vi "Periodic Tasks.vi"(8 "error in":errorcluster) -> ()   [LabVIEW 2018]
doc: "This VI runs in parallel to other tasks. It can contain as many user-defined periodic loops as you need. These can carry out PID or other sorts of timed response."
uses:
  <vilib>/Rock Robotics/WPI/ThirdParty/Sensors/navX/_TypeDefs/FRIC_navX_DeviceNumbersTypeDef.ctl
  <vilib>/Rock Robotics/WPI/Relay/WPI_RelayValue.ctl
  <vilib>/Rock Robotics/WPI/DriverStation/WPI_DriverStationRobotMode2.ctl
  <vilib>/Rock Robotics/WPI/Utilities/WPI_GetSetVariantRefNum.vi
  Robot Global Data.vi
  <vilib>/Rock Robotics/Network Tables/NT Write Number.vi
  <vilib>/Rock Robotics/WPI/ThirdParty/Phoenix-LabVIEW/Motor Controller/Get/CTRE_Phoenix_MotorController_GetQuadratureData.vi
  <vilib>/Rock Robotics/WPI/ThirdParty/Sensors/navX/_Processing Loop/FRIC_navX_Internal_Serial_ProcessingLoop.vi
panel:
  out "Largeur Vision":dbl
  out "Gauche Droite Vision":dbl
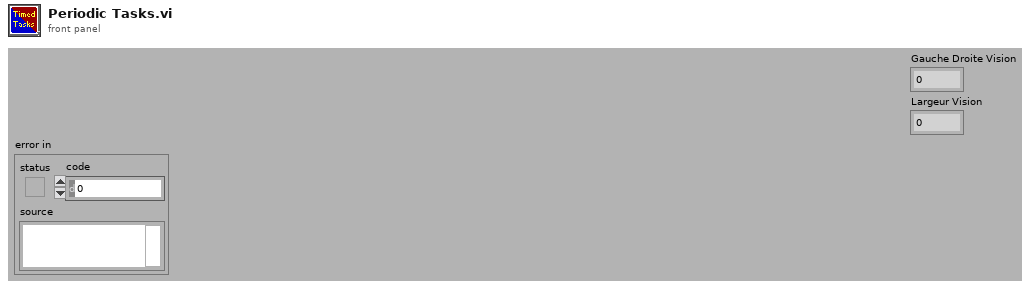
[diagram p1: front panel]
types:
  T1 = typedef "FRIC_navX_DeviceNumbersTypeDef.ctl" = enum16{"Dev0", "Dev1", "Dev2", "Dev3"}
  T2 = typedef "WPI_RelayDevRef.ctl" = cluster{"DevStatus":errorcluster, "Relay Channel":T3, "Relay Direction":T4}
  T3 = typedef "FPGA_DIORelayChannel.ctl" = enum8{"Relay 0", "Relay 1", "Relay 2", "Relay 3", "Invalid"}
  T4 = typedef "WPI_RelayDirection.ctl" = enum16{"Both directions", "Forward only", "Reverse only"}
  T5 = typedef "WPI_JoystickDevRef.ctl" = cluster{"Device":T6}
  T6 = typedef "WPI_JoystickDeviceEnum.ctl" = enum16{"USB 0", "USB 1", "USB 2", "USB 3", "USB 4", "USB 5"}
  T7 = typedef "WPI_RobotDriveDevRef.ctl" = cluster{"DevStatus":errorcluster, "Motors[]":T8[], "Square Inputs":bool, "Max Output":dbl}
  T8 = typedef "WPI_MotorControlDeviceRef.ctl" = cluster{"DeviceStatus":errorcluster, "Type":T9, "PWM":cluster{"PWM Channel":T10, "DeadBand":T11}, "CAN":cluster{"Device Number":u8, "SetOutput VI Ref":variant, "GetOutput VI Ref":variant, "Enable VI Ref":variant, "Disable VI Ref":variant, "Data":variant}, "Invert":bool, "DIO PWM":cluster{"PWM \"Enable\" Channel":T10, "DIOChannel":T12, "PWM Rate":dbl}}
  T9 = typedef "WPI_MotorControlType.ctl" = enum16{"PWM", "CAN", "DIO PWM"}
  T10 = typedef "FPGA_DIOPWMChannel.ctl" = enum8{"PWM 0", "PWM 1", "PWM 2", "PWM 3", "PWM 4", "PWM 5", "PWM 6", "PWM 7", "PWM 8", "PWM 9", "PWM MXP 0", "PWM MXP 1", "PWM MXP 2", "PWM MXP 3", "PWM MXP 4", "PWM MXP 5", "PWM MXP 6", "PWM MXP 7", "PWM MXP 8", "PWM MXP 9", "Invalid"}
  T11 = typedef "WPI_PWMDeadband.ctl" = cluster{"Name":string, "maxPositivePwm":i32, "minPositivePwm":i32, "centerPwm":i32, "maxNegativePwm":i32, "minNegativePwm":i32, "angularRange":u16}
  T12 = typedef "FPGA_DIOChannel.ctl" = enum8{"DIO 0", "DIO 1", "DIO 2", "DIO 3", "DIO 4", "DIO 5", "DIO 6", "DIO 7", "DIO 8", "DIO 9", "DIO MXP 0", "DIO MXP 1", "DIO MXP 2", "DIO MXP 3", "DIO MXP 4", "DIO MXP 5", "DIO MXP 6", "DIO MXP 7", "DIO MXP 8", "DIO MXP 9", "DIO MXP 10", "DIO MXP 11", "DIO MXP 12", "DIO MXP 13", "DIO MXP 14", "DIO MXP 15", "SPI Port CS1", "SPI Port CS2", "SPI Port CS3", "SPI Port MISO", "SPI Port MOSI", "Invalid"}
  T13 = cluster{"RelayDevRef":T2, "JoystickDevRef":T5, "RobotDriveDevRef":T7, "PhoenixMotorControlDevRef":T8, "PhoenixMotorControlDevRef":T8, "PhoenixMotorControlDevRef":T8, "PhoenixMotorControlDevRef":T8}
  T14 = typedef "WPI_DriverStationRobotMode2.ctl" = enum16{"Autonomous Disabled", "Autonomous Enabled", "Teleop Disabled", "Teleop Enabled", "Disconnected", "Finish", "Test Disabled", "Test Enabled", "Emergency Stopped"}
  T15 = typedef "WPI_RelayValue.ctl" = enum16{"Off", "On", "Forward", "Reverse"}
  T16 = cluster{"Yaw":dbl, "Roll":dbl, "Pitch":dbl, "Heading":dbl, "Fused Heading":dbl}
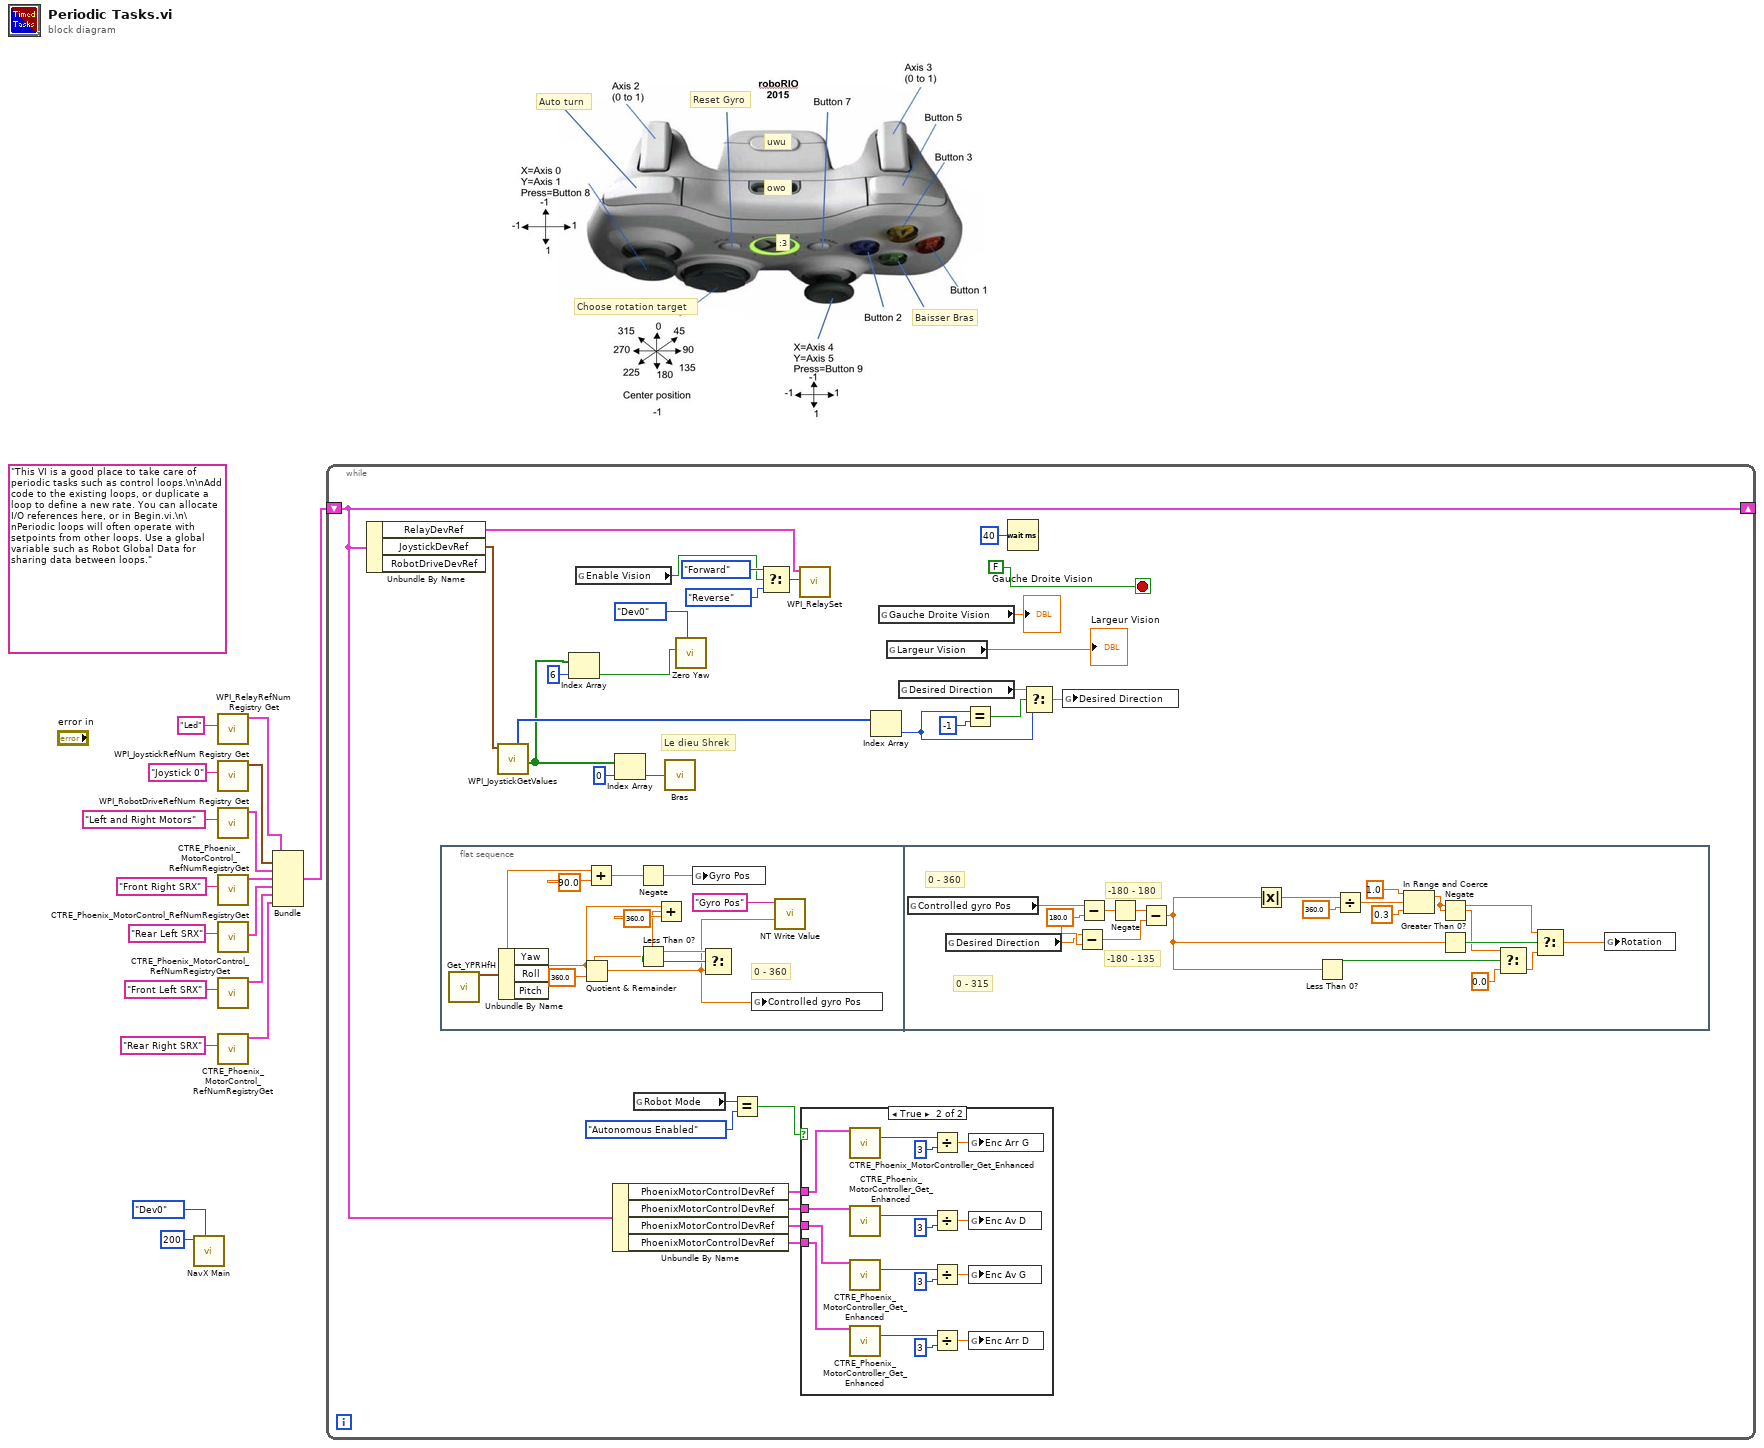
[diagram p0: block diagram]
diagram:
  (unwired) "This VI is a good place to take care of periodic tasks such as control loops.\n\nAdd code to the existing loops, or duplicate a loop to define a new rate. You can allocate I/O references here, or in Begin.vi.\n\nPeriodic loops will often operate with setpoints from other loops. Use a global variable such as Robot Global Data for sharing data between loops."
  # "Baisser Bras"
  # "Choose rotation target"
  # "Auto turn"
  # "Reset Gyro"
  # ":3"
  # "owo"
  # "uwu"
  n1 = call-poly <vilib>:"NavX Main.vi"("Device Number"=FRIC_navX_DeviceNumbersTypeDef."Dev0", "Rate (4Hz-200Hz)"=u8 200) -> ()  [unwired: 10 in]
  n2 = call <vilib>:"WPI_RelayRefNum Registry Get.vi"("refnum name"="Led") -> ("RelayDevRef"=w11:T2)  [unwired: 9 in, 1 out]
  n3 = call <vilib>:"WPI_JoystickRefNum Registry Get.vi"("refnum name"="Joystick 0") -> ("JoystickDevRef"=w15:T5)  [unwired: 1 in, 9 out]
  n4 = call <vilib>:"WPI_RobotDriveRefNum Registry Get.vi"("refnum name"="Left and Right Motors") -> ("RobotDriveDevRef"=w14:T7)  [unwired: 1 in, 9 out]
  n5 = call <vilib>:"CTRE_Phoenix_MotorControl_RefNumRegistryGet.vi"("refnum name"="Front Right SRX") -> ("PhoenixMotorControlDevRef"=w6:T8)  [unwired: 9 in, 1 out]
  n6 = call <vilib>:"CTRE_Phoenix_MotorControl_RefNumRegistryGet.vi"("refnum name"="Rear Left SRX") -> ("PhoenixMotorControlDevRef"=w5:T8)  [unwired: 9 in, 1 out]
  n7 = call <vilib>:"CTRE_Phoenix_MotorControl_RefNumRegistryGet.vi"("refnum name"="Front Left SRX") -> ("PhoenixMotorControlDevRef"=w4:T8)  [unwired: 9 in, 1 out]
  n8 = call <vilib>:"CTRE_Phoenix_MotorControl_RefNumRegistryGet.vi"("refnum name"="Rear Right SRX") -> ("PhoenixMotorControlDevRef"=w3:T8)  [unwired: 9 in, 1 out]
  n9 = Bundle("RelayDevRef"=w11, "JoystickDevRef"=w15, "RobotDriveDevRef"=w14, "PhoenixMotorControlDevRef"=w6, "PhoenixMotorControlDevRef"=w5, "PhoenixMotorControlDevRef"=w4, "PhoenixMotorControlDevRef"=w3) -> (w13:T13)  [unwired: 1 out]
  n10 = while {
    shift-right: [w23] -> _
    shift-left: w13 -> [w23]
    stop <- FALSE stop-if-true
    # "Le dieu Shrek"
    n11 = Unbundle By Name(w23) -> ("RelayDevRef"=w29:T2, "JoystickDevRef"=w45:T5)  [unwired: 1 out]
    n12 = flat-sequence {
      frame #0 {
        # "0 - 360"
        n13 = call <vilib>:"Get_YPRHfH.vi"() -> ("YRPHfH"=w59:T16)  [unwired: 11 in]
        n14 = Unbundle By Name(w59) -> ("Yaw"=w48:dbl)  [unwired: 2 out]
        n15 = Quotient & Remainder(x=w48, y=360.0) -> (x-y*floor(x/y)=w54:dbl)  [unwired: 1 out]
        n16 = Add(x=w48, y=90.0) -> (x+y=w49:dbl)
        n17 = Negate(x=w49) -> (-x=w51:dbl)
        n18 = Less Than 0?(x=w54) -> (x < 0?=w55:bool)
        n19 = Add(x=w54, y=360.0) -> (x+y=w53:dbl)
        n20 = global write "Robot Global Data.vi" "Gyro Pos"(w51) -> ()
        n21 = Select(t=w53, s=w55, f=w54) -> (s? t:f=w52:dbl)
        n22 = global write "Robot Global Data.vi" "Controlled gyro Pos"(w52) -> ()
        n23 = call-poly <vilib>:"NT Write Value.vi"("Numeric"=w52, "Name"="Gyro Pos") -> ()  [unwired: 9 in, 1 out]
      }
      frame #1 {
        w61 = 180.0 ("y")
        # "-180 - 135"
        # "-180 - 180"
        # "0 - 315"
        # "0 - 360"
        n24 = global read "Robot Global Data.vi" "Controlled gyro Pos"() -> (w65:dbl)
        n25 = global read "Robot Global Data.vi" "Desired Direction"() -> (w60:dbl)
        n26 = Subtract(x=w60, y=w61) -> (x-y=w62:dbl)
        n27 = Subtract(x=w65, y=w61) -> (x-y=w64:dbl)
        n28 = Negate(x=w64) -> (-x=w63:dbl)
        n29 = Subtract(x=w63, y=w62) -> (x-y=w67:dbl)
        n30 = Absolute Value(x=w67) -> (abs(x)=w78:dbl)
        n31 = Less Than 0?(x=w67) -> (x < 0?=w69:bool)
        n32 = Divide(x=w78, y=360.0) -> (x/y=w76:dbl)
        n33 = In Range and Coerce(upper limit=1.0, x=w76, lower limit=0.3) -> (coerced(x)=w71:dbl)  [unwired: 1 out]
        n34 = Negate(x=w71) -> (-x=w70:dbl)
        n35 = Greater Than 0?(x=w67) -> (x > 0?=w72:bool)
        n36 = Select(t=w70, s=w69, f=0.0) -> (s? t:f=w73:dbl)
        n37 = Select(t=w71, s=w72, f=w73) -> (s? t:f=w66:dbl)
        n38 = global write "Robot Global Data.vi" "Rotation"(w66) -> ()
      }
    }
    n39 = call <vilib>:"WPI_JoystickGetValues.vi"("JoystickDevRef"=w45) -> ("Buttons"=w36:bool[], "POVs"=w44:i16[])  [unwired: 6 in, 3 out]
    n40 = Index Array(array=w36, index=6) -> (element=w34:bool)
    n41 = global read "Robot Global Data.vi" "Enable Vision"() -> (w28:bool)
    n42 = Unbundle By Name(w23) -> ("PhoenixMotorControlDevRef"=w22:T8, "PhoenixMotorControlDevRef"=w21:T8, "PhoenixMotorControlDevRef"=w20:T8, "PhoenixMotorControlDevRef"=w19:T8)
    n43 = Index Array(array=w36, index=0) -> (element=w38:bool)
    n44 = global read "Robot Global Data.vi" "Robot Mode"() -> (w24:T14)
    n45 = call "Bras.vi"("Commande"=w38) -> ()
    n46 = call <vilib>:"Zero Yaw.vi"("Device Number"=FRIC_navX_DeviceNumbersTypeDef."Dev0", "Zero"=w34) -> ()  [unwired: 10 in]
    n47 = Equal?(x=w24, y=WPI_DriverStationRobotMode2."Autonomous Enabled") -> (x = y?=w18:bool)
    n48 = Select(t=WPI_RelayValue."Forward", s=w28, f=WPI_RelayValue."Reverse" ("RelayValue")) -> (s? t:f=w30:T15)
    n49 = call <vilib>:"WPI_RelaySet.vi"("RelayValue"=w30, "RelayDevRef"=w29) -> ()  [unwired: 8 in, 2 out]
    n50 = case shown="True" w18 {
      tunnel: w22 -> [_ w94]
      tunnel: w21 -> [_ w93]
      tunnel: w20 -> [_ w92]
      tunnel: w19 -> [_ w91]
      frame False {
      }
      frame True {
        n51 = call-poly <vilib>:"CTRE_Phoenix_MotorController_Get_Enhanced.vi"("PhoenixMotorControlDevRef"=w94) -> ("Quadrature Position"=w89:i32)  [unwired: 11 in, 3 out]
        n52 = call-poly <vilib>:"CTRE_Phoenix_MotorController_Get_Enhanced.vi"("PhoenixMotorControlDevRef"=w93) -> ("Quadrature Position"=w90:i32)  [unwired: 11 in, 3 out]
        n53 = call-poly <vilib>:"CTRE_Phoenix_MotorController_Get_Enhanced.vi"("PhoenixMotorControlDevRef"=w92) -> ("Quadrature Position"=w87:i32)  [unwired: 11 in, 3 out]
        n54 = call-poly <vilib>:"CTRE_Phoenix_MotorController_Get_Enhanced.vi"("PhoenixMotorControlDevRef"=w91) -> ("Quadrature Position"=w88:i32)  [unwired: 11 in, 3 out]
        n55 = Divide(x=w89, y=3) -> (x/y=w79:dbl)
        n56 = Divide(x=w90, y=3) -> (x/y=w80:dbl)
        n57 = Divide(x=w87, y=3) -> (x/y=w81:dbl)
        n58 = Divide(x=w88, y=3) -> (x/y=w82:dbl)
        n59 = global write "Robot Global Data.vi" "Enc Arr G"(w79) -> ()
        n60 = global write "Robot Global Data.vi" "Enc Av D"(w80) -> ()
        n61 = global write "Robot Global Data.vi" "Enc Av G"(w81) -> ()
        n62 = global write "Robot Global Data.vi" "Enc Arr D"(w82) -> ()
      }
    }
    n63 = Index Array(array=w44) -> (element=w39:i16)  [unwired: 1 in]
    n64 = global read "Robot Global Data.vi" "Gauche Droite Vision"() -> (→"Gauche Droite Vision":dbl)
    n65 = global read "Robot Global Data.vi" "Largeur Vision"() -> (→"Largeur Vision":dbl)
    n66 = global read "Robot Global Data.vi" "Desired Direction"() -> (w41:dbl)
    n67 = Equal?(x=w39, y=i16 -1) -> (x = y?=w42:bool)
    n68 = Wait (ms)(milliseconds to wait=u32 40) -> ()  [unwired: 1 out]
    n69 = Select(t=w41, s=w42, f=w39) -> (s? t:f=w40:dbl)
    n70 = global write "Robot Global Data.vi" "Desired Direction"(w40) -> ()
  }
